vi "DBVar ClassificationTypeInput.vi"(1 "type wired?":bool, 2 "Type":variant) -> (0 "type  classification":T1(ring))   [LabVIEW 2020, in "NI_DB Variant To Data Support.lvlib"]
uses:
  <vilib>/addons/database/_DB Variant To Data/NI_DB Variant To Data Support.lvlib
  <vilib>/Utility/VariantDataType/Type.ctl
  <vilib>/Utility/VariantDataType/VariantType.lvlib
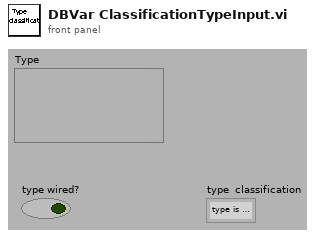
[diagram p1: front panel]
types:
  T1 = enum16{"type is cluster", "type is 1D array of scalar type", "type is 1D array of cluster type", "type is 2D array", "type is others", "type is unwired"}
  T2 = typedef "VariantType.lvlib/Type.ctl" = enum8{"Invalid Type", "Void", "I8", "I16", "I32", "I64", "U8", "U16", "U32", "U64", "Single Float", "Double Float", "Extended Float", "Single Complex", "Double Complex", "Extended Complex", "Enum U8", "Enum U16", "Enum U32", "Enum U64", "Single Float With Unit", "Double Float With Unit", "Extended Float With Unit", "Single Complex with Unit", "Double Complex with Unit", "Extended Complex with Unit", "Boolean", "String", "Path", "Picture", "Tag", "Array", "Cluster", "Variant", "LV Variant", "Waveform", "Timestamp", "Digital Waveform", "Digital Data", "ExpressData", "Refnum", "External Data", "VI", "Poly VI", "LabVIEW Class Instance", "Fixed Point"}
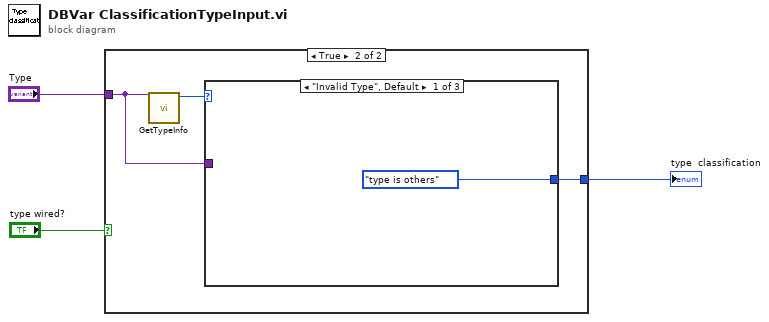
[diagram p0: block diagram]
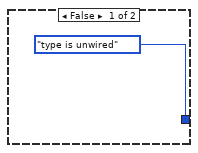
[diagram p2: hidden frame]
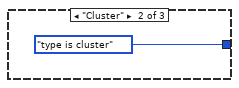
[diagram p3: hidden frame]
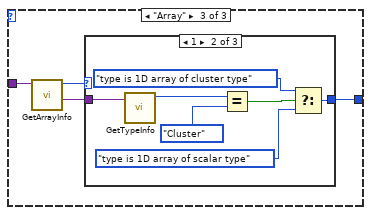
[diagram p4: hidden frame]
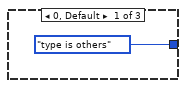
[diagram p5: hidden frame]
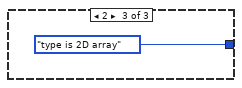
[diagram p6: hidden frame]
diagram:
  n1 = case shown="True" "type wired?" {
    tunnel: "Type" -> [_ w5]
    tunnel: [T1."type is unwired" ("type  classification") w6] -> w1
    frame False {
    }
    frame True {
      n2 = call <vilib>:"GetTypeInfo.vi"("Variant"=w5) -> ("Type Enum"=w7:T2)  [unwired: 1 in, 9 out]
      n3 = case shown="\"Invalid Type\", Default" w7 {
        tunnel: [T1."type is others" ("type  classification") T1."type is cluster" ("type  classification") w10] -> w6
        tunnel: w5 -> [_ _ w11]
        frame "Invalid Type", Default {
        }
        frame "Cluster" {
        }
        frame "Array" {
          n4 = call <vilib>:"GetArrayInfo.vi"("Variant"=w11) -> ("ArrayElement"=w13:variant, "NDims"=w12:i32)  [unwired: 7 in, 2 out]
          n5 = case shown="1" w12 {
            tunnel: [T1."type is others" ("type  classification") w17 T1."type is 2D array" ("type  classification")] -> w10
            tunnel: w13 -> [_ w21 _]
            frame 0, Default {
            }
            frame 1 {
              n6 = call <vilib>:"GetTypeInfo.vi"("Variant"=w21) -> ("Type Enum"=w20:T2)  [unwired: 1 in, 9 out]
              n7 = Equal?(x=w20, y=Type."Cluster" ("Type Enum")) -> (x = y?=w18:bool)
              n8 = Select(t=T1."type is 1D array of cluster type" ("type  classification"), s=w18, f=T1."type is 1D array of scalar type" ("type  classification")) -> (s? t:f=w17:T1)
            }
            frame 2 {
            }
          }
        }
      }
    }
  }
  "type  classification" <- w1
